vi "Visa Open wrapper.vi"(11 "VISA resource":refnum<visa-resource-name>) -> (3 "VISA resource name out":refnum<visa-resource-name>)   [LabVIEW 2017]
uses:
  <vilib>/Instr/_visa.llb/VISA Open Access Mode.ctl
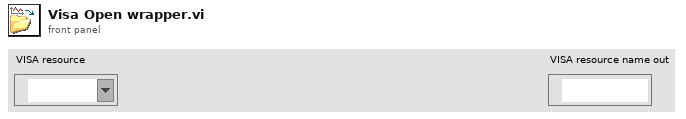
[diagram p1: front panel]
types:
  T1 = typedef "VISA Open Access Mode.ctl" = u32
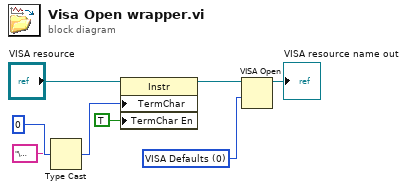
[diagram p0: block diagram]
diagram:
  w7 = T1 0 items=["VISA Defaults"=0, "Exclusive Lock"=1, "Load Configured Settings"=4] ("Access Mode")
  n1 = Type Cast(type=u8 0, x="\u0003") -> (*(type *) &x=w5:u8)
  n2 = property class="Instr"(reference="VISA resource", "TermChar"=w5, "TermChar En"=TRUE) -> (reference out=w8:refnum<visa-resource-name>)  [unwired: 1 in, 1 out]
  n3 = VISA Open(access mode=w7, VISA resource name=w8) -> (VISA resource name=→"VISA resource name out":refnum<visa-resource-name>)  [unwired: 3 in, 1 out]
